vi "createPythonInstance.vi"(0 "reference in":refnum<class "File Controller.lvclass">, 5 "error in (no error)":errorcluster) -> (14 "reference out":refnum<class "File Controller.lvclass">, 19 "error out":errorcluster)   [LabVIEW 2014, in "File Controller.lvclass"]
uses:
  File Controller.lvclass
  APP/python_class/python.lvclass
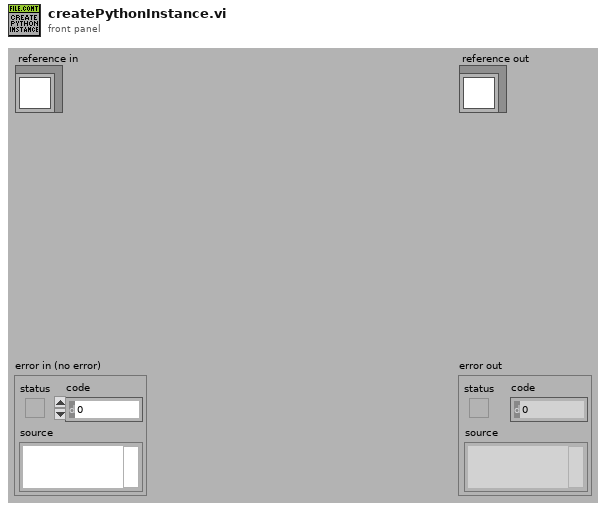
[diagram p1: front panel]
types:
  T1 = typedef "File Controller.lvclass/ObjectAttributesRef.ctl" = refnum<data-value>
  T2 = typedef "File Controller.lvclass/ObjectAttributes.ctl" = cluster{"MyAttribute":dbl, "excelFile_refs":refnum<class "excelFile.lvclass">[], "filePaths":path[], "outlookTemplatePaths":path[], "attachmentTemplatePaths":path[], "configFilePath":path, "not_setting":bool[], "python_ref":refnum<class "python.lvclass">}
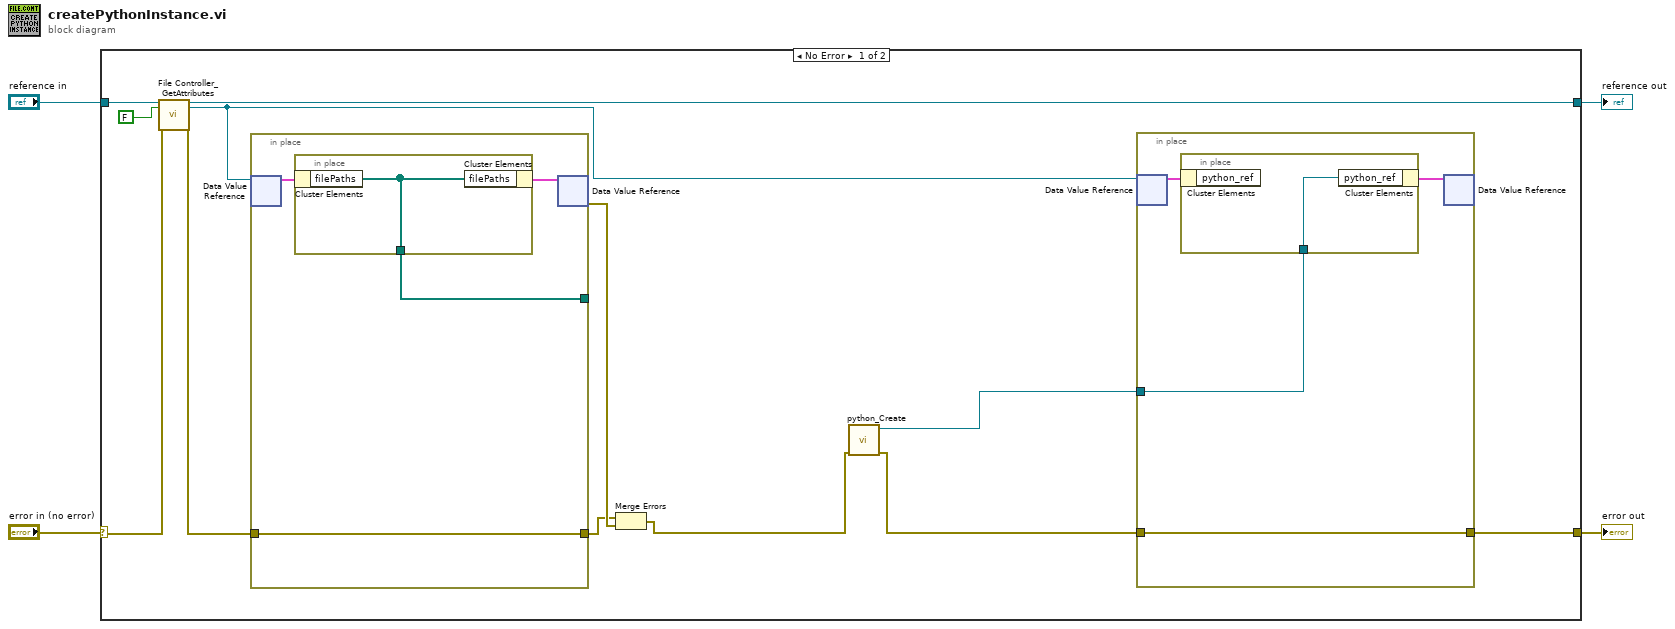
[diagram p0: block diagram]
diagram:
  n1 = case shown="No Error" "error in (no error)" {
    selector: "error in (no error)" -> [w12 w28]
    tunnel: [w9 w28] -> w3
    tunnel: [w10 w27] -> w1
    tunnel: "reference in" -> [w14 w27]
    frame No Error {
      n2 = call "File Controller_GetAttributes.vi"("reference in"=w14, "return data? (T)"=FALSE, "error in (no error)"=w12) -> ("reference out"=w10:refnum<class "File Controller.lvclass">, "attributes ref"=w8:T1, "error out"=w11:errorcluster)  [unwired: 13 in, 1 out]
      n3 = in-place {
        in-place-border: w11 -> [w23]
        in-place-border: [w23] -> w15
        in-place-border: [w22] -> _
        n4 = in-place-dvr #1(w8) -> (w24:T2)  [unwired: 1 out]
        n5 = in-place {
          in-place-border: [w26] -> w22
          n6 = in-place-cluster #2(w24) -> ("filePaths"=w26:path[])
          n7 = in-place-cluster #2("filePaths"=w26) -> (w25:T2)
        }
        n8 = in-place-dvr #1(w25) -> (w16:errorcluster)  [unwired: 1 out]
      }
      n9 = Merge Errors(w15, w16) -> (w7:errorcluster)
      n10 = call "python_Create.vi"("error in (no error)"=w7) -> ("error out"=w6:errorcluster, "reference out"=w5:refnum<class "python.lvclass">)  [unwired: 9 in]
      n11 = in-place {
        in-place-border: w6 -> [w18]
        in-place-border: [w18] -> w9
        in-place-border: w5 -> [w17]
        n12 = in-place-dvr #3(w8) -> (w19:T2)  [unwired: 1 out]
        n13 = in-place {
          in-place-border: w17 -> [w21]
          n14 = in-place-cluster #4(w19) -> ()  [unwired: 1 out]
          n15 = in-place-cluster #4("python_ref"=w21) -> (w20:T2)
        }
        n16 = in-place-dvr #3(w20) -> ()  [unwired: 2 out]
      }
    }
    frame Error {
    }
  }
  "error out" <- w3
  "reference out" <- w1
